vi "hmi3.vi"() -> ()   [LabVIEW 2017]
doc: "Demonstrates how to write and receive CAN frames via the Network Interface on the same port. \n\nTo write and receive frames via the Network Interface:\n- select the CAN Network Interface (i.e. CAN0, CAN1, etc.)\n- select the Baud Rate\n- run the VI\n- press the write button to write frames to the can bus\n\nEnable RTR Button to send a Remote Transmission Request or to simply send an empty Frame to request an Answer Frame from a connected device.\n\nEnable Extended Button to write extended Identifier Format. This is done by setting the 30th bit to enable extended format with the driver."
uses:
  <vilib>/nican/nican.llb/ncNetAttr.ctl
panel:
  in  "InitForceUpdate?":bool
  in  "IND2":bool
  in  "IND1":bool
  out "Data":u8[](array[numeric])
  out "Heartbeat":u16 format="%04x"
  in  "interface":string(combo)="CAN0" caption="Interface"
  in  "shutdown":bool
  # "PRESS AND HOLD"
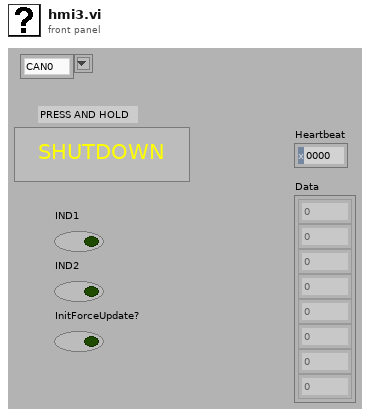
[diagram p1: front panel]
types:
  T1 = typedef "ncNetAttr.ctl" = cluster{"Start On Open":enum32{"FALSE", "TRUE"}, "Baud Rate":u32, "Read Queue Length":u32, "Write Queue Length":u32, "Standard Comparator":u32, "Standard Mask":u32, "Extended Comparator":u32, "Extended Mask":u32}
  T2 = typedef "xobjhandle.ctl" = u32
  T3 = typedef "CanFrameTimed.ctl" = cluster{"Timestamp":dbl, "ArbitrationId":u32, "IsRemote":u8, "DataLength":u8, "Data":u8[]}
  T4 = cluster{dbl, u32, "IsRemote":u8, "DataLength":u8, u8[]}
  T5 = cluster{dbl, u32, "IsRemote":u8, "DataLength":u8, u8[]}[]
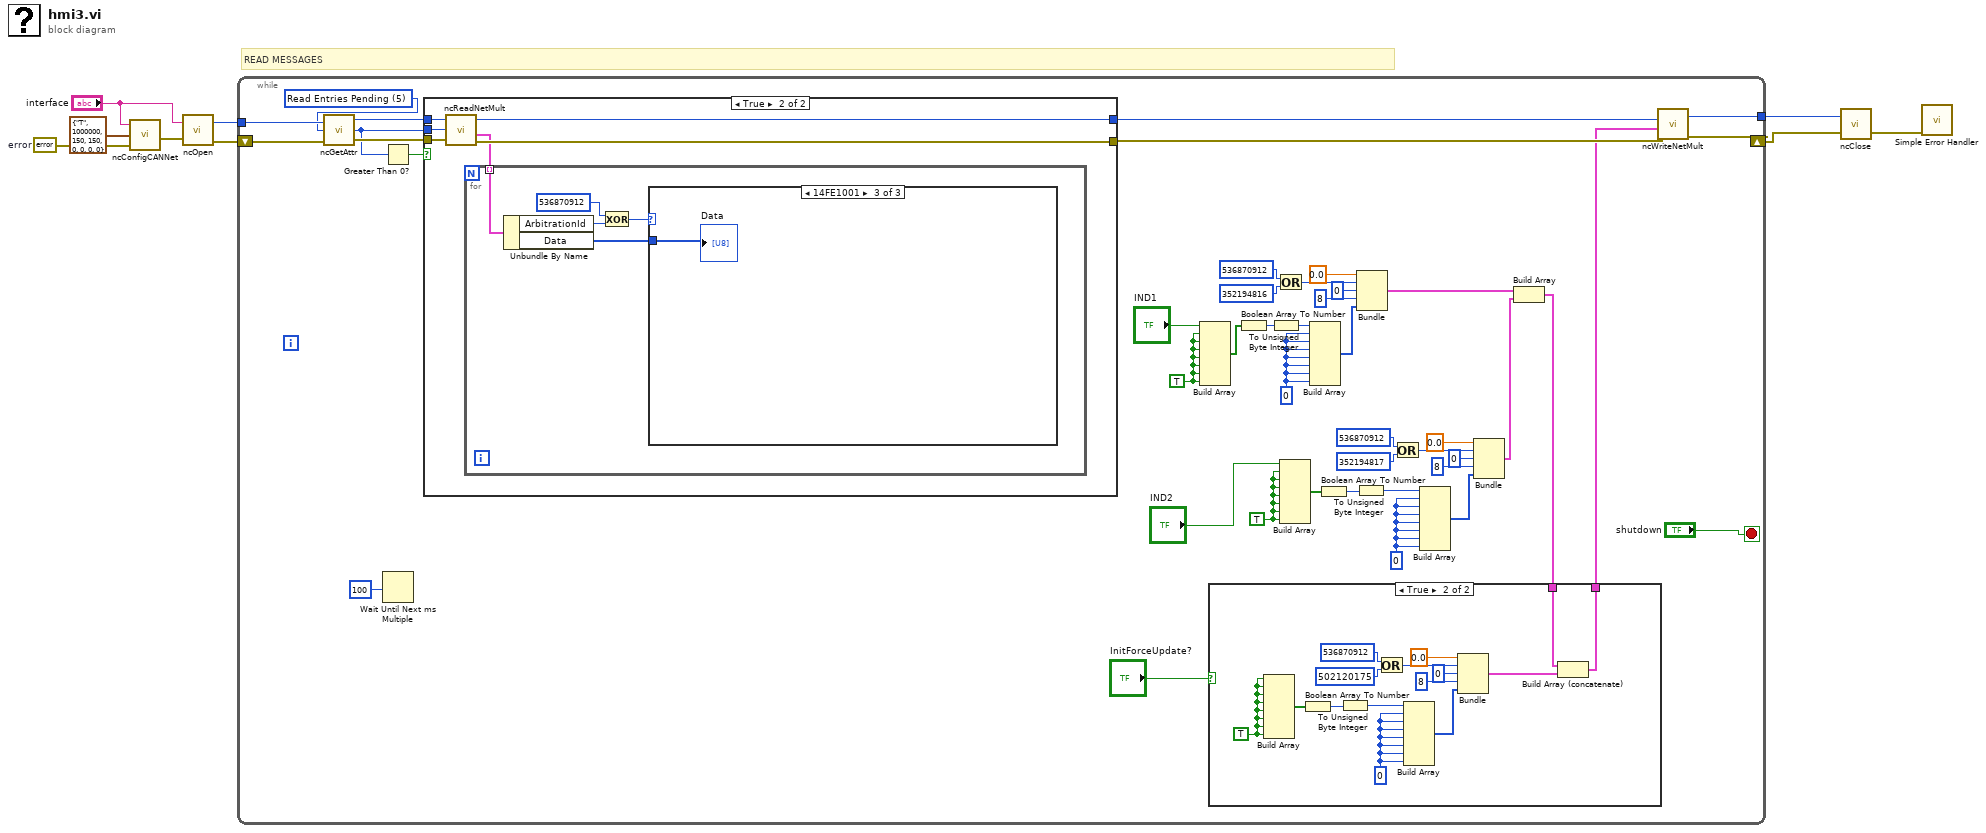
[diagram p0: block diagram]
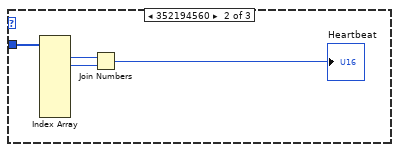
[diagram p5: hidden frame]
diagram:
  w5 = errorcluster {"status"=FALSE, "code"=0, "source"=""}  # error
  # "READ MESSAGES"
  n1 = call <vilib>:"ncConfigCANNet.vi"("Error in"=w5, "CAN Network Interface Config"=T1 {"Start On Open"=enum."TRUE", "Baud Rate"=1000000, "Read Queue Length"=150, "Write Queue Length"=150, "Standard Comparator"=0, "Standard Mask"=0, "Extended Comparator"=0, "Extended Mask"=0}, "ObjName"="interface") -> ("Error out"=w6:errorcluster)  [unwired: 2 in]
  n2 = call <vilib>:"ncOpen.vi"("Error in"=w6, "ObjName"="interface") -> ("Error out"=w9:errorcluster, "ObjHandle out"=w7:T2)
  n3 = while {
    tunnel: w7 -> [w47]
    tunnel: [w52] -> w2
    shift-right: [w53] -> w1
    shift-left: w9 -> [w46]
    stop <- "shutdown" stop-if-true
    w21 = TRUE ("element")
    w23 = TRUE ("element")
    w26 = u8 0
    w34 = u8 0
    w43 = u32 5 items=["(reserved)", "Protocol Version", "Software Version", "Object State", "(reserved)", "Read Entries Pending", "Write Entries Pending", "ReadMult Size for Notification", "Listen Only?", "Self Reception?", "Transmit Error Counter", "Receive Error Counter", "Single Shot Transmit?", "Series 2 Filter Mode", "Series 2 Mask", "Series 2 Comparator", "Serial Number", "Form Factor", "Series", "Transceiver Type", "Interface Number", "Series 2 Error/Arb Capture", "Transceiver Mode", "Transceiver External Outputs", "Transceiver External Inputs", "Start Trigger Behavior", "Log Comm Warnings", "User RTSI Frame", "Transmit Mode", "Log Start Trigger?", "Timestamp Format", "Master Timebase Rate", "Virtual Bus Timing"] ("AttrId")
    n4 = call <vilib>:"ncGetAttr.vi"("Error in"=w46, "AttrId"=w43, "ObjHandle in"=w47) -> ("Error out"=w51:errorcluster, "AttrValue"=w48:u32, "ObjHandle out"=w50:T2)
    n5 = Greater Than 0?(x=w48) -> (x > 0?=w49:bool)
    n6 = Wait Until Next ms Multiple(millisecond multiple=u32 100) -> ()  [unwired: 1 out]
    n7 = case shown="True" w49 {
      tunnel: [w70 w77] -> w44
      tunnel: [w71 w76] -> w45
      tunnel: w48 -> [_ w75]
      tunnel: w51 -> [w70 w74]
      tunnel: w50 -> [w71 w73]
      frame False {
      }
      frame True {
        n8 = call <vilib>:"ncReadNetMult.vi"("ObjHandle in"=w73, "Requested Number of Frames"=w75, "Error in"=w74) -> ("ObjHandle out"=w76:T2, "Data"=w72:T3[], "Error out"=w77:errorcluster)  [unwired: 1 out]
        n9 = for {
          tunnel: w72 -> [w82] mode=indexing
          n10 = Unbundle By Name(w82) -> ("ArbitrationId"=w80:u32, "Data"=w78:u8[])
          n11 = Exclusive Or(1:w80, 2:u32 536870912 ("y")) -> (0:w79:u32)
          n12 = case shown="14FE1001" w79 {
            tunnel: w78 -> [_ w86 w87]
            frame Default {
            }
            frame 352194560 {
              n13 = Index Array(array=w86) -> (element #1=w84:u8, element #2=w85:u8)  [unwired: 8 in, 6 out]
              n14 = Join Numbers(hi=w84, lo=w85) -> ((hi.lo)=→"Heartbeat":u16)
            }
            frame 352194561 {
              "Data" <- w87
            }
          }
        }
      }
    }
    n15 = Build Array("IND1", w23, w23, w23, w23, w23, w23, w23) -> (w17:bool[])
    n16 = Boolean Array To Number(Boolean array=w17) -> (number=w19:u32)
    n17 = To Unsigned Byte Integer(number=w19) -> (unsigned 8bit integer=w18:u8)
    n18 = Or(x=u32 536870912 ("y"), y=u32 352194816) -> (x .or. y?=w32:u32)
    n19 = Build Array("IND2", w21, w21, w21, w21, w21, w21, w21) -> (w22:bool[])
    n20 = Build Array(w18, w26, w26, w26, w26, w26, w26, w26) -> (w28:u8[])
    n21 = Boolean Array To Number(Boolean array=w22) -> (number=w15:u32)
    n22 = To Unsigned Byte Integer(number=w15) -> (unsigned 8bit integer=w16:u8)
    n23 = Bundle(0.0, w32, "IsRemote"=u8 0, "DataLength"=u8 8, w28) -> (w25:T4)  [unwired: 1 in]
    n24 = Or(x=u32 536870912 ("y"), y=u32 352194817) -> (x .or. y?=w40:u32)
    n25 = Build Array(w16, w34, w34, w34, w34, w34, w34, w34) -> (w36:u8[])
    n26 = Bundle(0.0, w40, "IsRemote"=u8 0, "DataLength"=u8 8, w36) -> (w13:T4)  [unwired: 1 in]
    n27 = Build Array(w25, w13) -> (w12:T5)
    n28 = case shown="True" "InitForceUpdate?" {
      tunnel: w12 -> [w54 w58]
      tunnel: [w54 w56] -> w11
      frame False {
      }
      frame True {
        w55 = TRUE ("element")
        w66 = u8 0
        n29 = Build Array(w55, w55, w55, w55, w55, w55, w55, w55) -> (w67:bool[])
        n30 = Boolean Array To Number(Boolean array=w67) -> (number=w69:u32)
        n31 = To Unsigned Byte Integer(number=w69) -> (unsigned 8bit integer=w68:u8)
        n32 = Or(x=u32 536870912 ("y"), y=u32 502120175) -> (x .or. y?=w60:u32)
        n33 = Build Array(w68, w66, w66, w66, w66, w66, w66, w66) -> (w64:u8[])
        n34 = Bundle(0.0, w60, "IsRemote"=u8 0, "DataLength"=u8 8, w64) -> (w57:T4)  [unwired: 1 in]
        n35 = Build Array (concatenate)(w58, w57) -> (w56:T5)
      }
    }
    n36 = call <vilib>:"ncWriteNetMult.vi"("Error in"=w44, "Data"=w11, "ObjHandle in"=w45) -> ("Error out"=w53:errorcluster, "ObjHandle out"=w52:T2)  [unwired: 7 in]
  }
  n37 = call <vilib>:"ncClose.vi"("Error in"=w1, "ObjHandle in"=w2) -> ("Error out"=w3:errorcluster)  [unwired: 1 in]
  n38 = call <vilib>:"Simple Error Handler.vi"("error in (no error)"=w3) -> ()  [unwired: 4 in, 5 out]
